vi "Send Message (Text-based).vi"(8 "error in (no error)":errorcluster, 10 "Message":string, 11 "MSOX6004 in":refnum<class "MSOX6004.lvclass">) -> (0 "error out":errorcluster, 3 "MSOX6004 out":refnum<class "MSOX6004.lvclass">)   [LabVIEW 2018, in "MSOX6004.lvlib" / "MSOX6004.lvclass"]
uses:
  MSOX6004.lvclass
  MSOX6004.lvclass/MSOX6004.ctl
  <instrlib>/Keysight InfiniiVision/Keysight InfiniiVision.lvlib
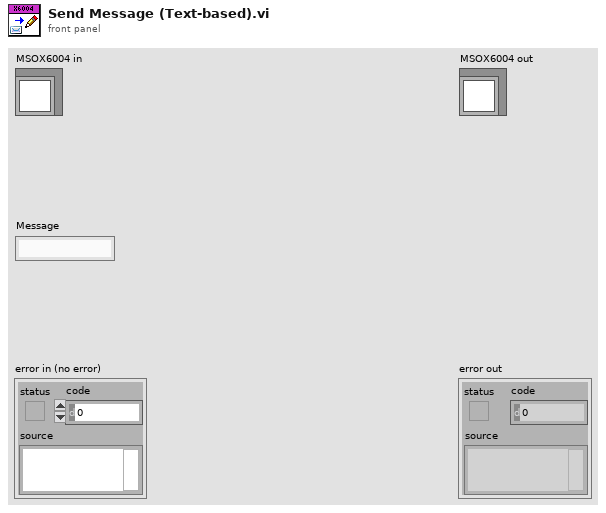
[diagram p1: front panel]
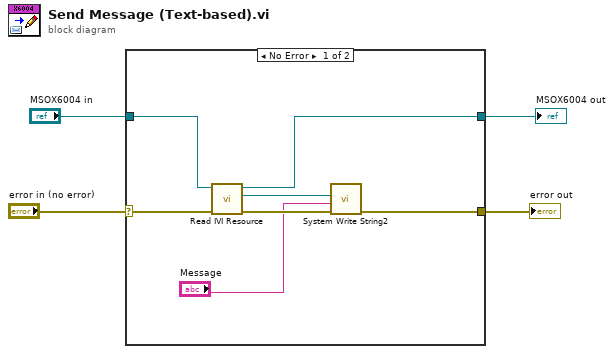
[diagram p0: block diagram]
diagram:
  n1 = case shown="No Error" "error in (no error)" {
    selector: "error in (no error)" -> [w5 w12]
    tunnel: "MSOX6004 in" -> [w8 w13]
    tunnel: [w7 w13] -> w3
    tunnel: [w6 w12] -> w2
    frame No Error {
      n2 = call "Read IVI Resource.vi"("error in (no error)"=w5, "MSOX6004 in"=w8) -> ("error out"=w10:errorcluster, "IVI Resource"=w11:refnum<k15>, "MSOX6004 out"=w7:refnum<class "MSOX6004.lvclass">)  [unwired: 7 in]
      n3 = call <instrlib>:"System Write String2.vi"("error in (no error)"=w10, "Data"="Message", "instrument handle"=w11) -> ("error out"=w6:errorcluster)  [unwired: 7 in, 1 out]
    }
    frame Error {
    }
  }
  "error out" <- w2
  "MSOX6004 out" <- w3
